vi "Do snap rpc cmd.vi"(8 "error in (no error)":errorcluster, 9 "Custom Command":string, 10 "Radio Address":string) -> (0 "error out":errorcluster, 1 "Cmd":string, 2 "standard error":string, 3 "trimmed string":string, 4 "return code":i32, 5 "standard output":string, 6 "Data item 1":string, 7 "Real volts":dbl, 11 "State":bool)   [LabVIEW 2013]
uses:
  1000336 func types.ctl
panel:
  in  "Function":T1
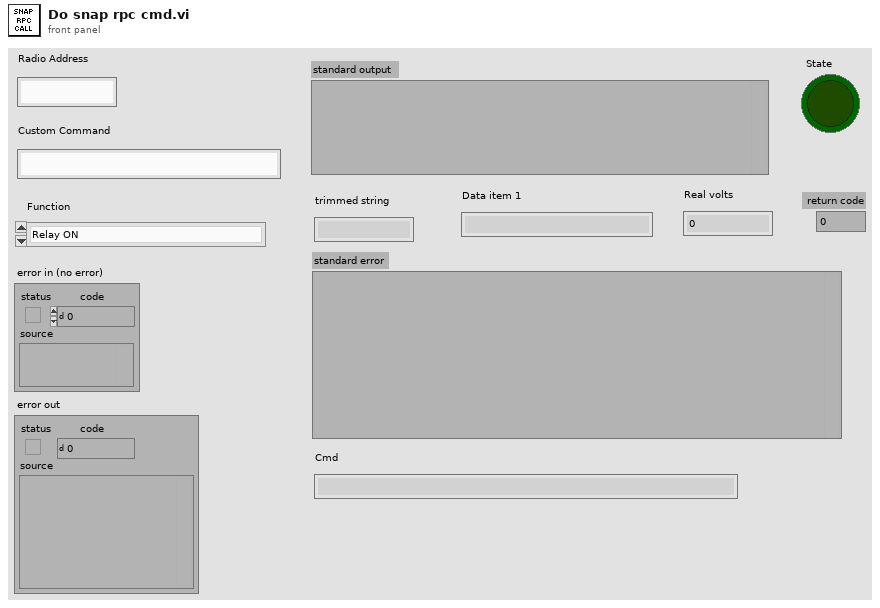
[diagram p1: front panel]
types:
  T1 = typedef "1000336 func types.ctl" = enum16{"Relay ON", "Relay OFF", "Override switch ON?", "Override switch OFF?", "Meas_vdc", "Meas_24v", "Meas_3.3v", "Blue led ON", "Blue led OFF", "Red led ON", "Red led OFF", "Green led ON", "Green led OFF", "Auto led ON", "Auto led OFF", "Custom cmd", "Get relay state", "Get major software version", "Get minor software version", "Get build version"}
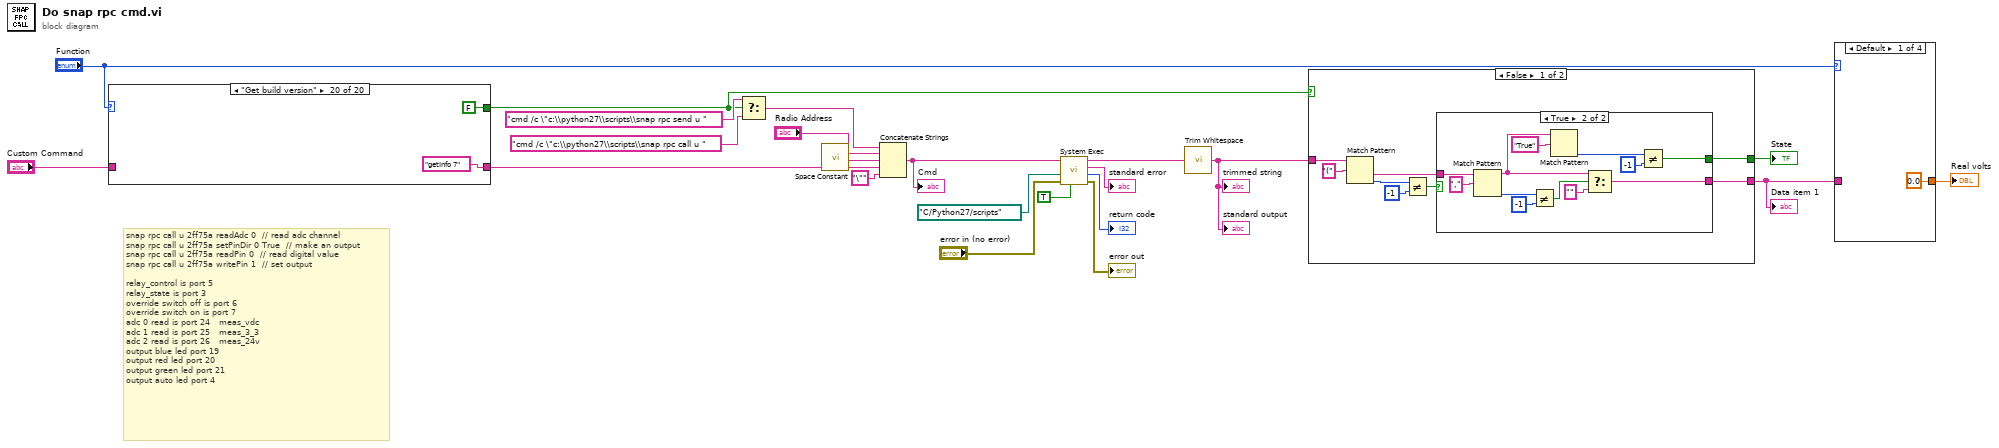
[diagram p0: block diagram]
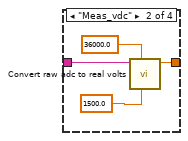
[diagram p2: hidden frame]
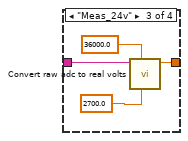
[diagram p3: hidden frame]
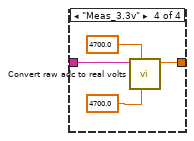
[diagram p4: hidden frame]
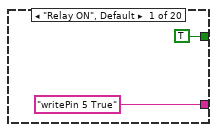
[diagram p5: hidden frame]
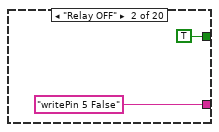
[diagram p6: hidden frame]
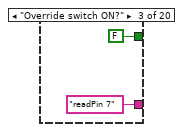
[diagram p7: hidden frame]
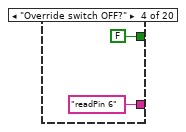
[diagram p8: hidden frame]
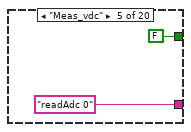
[diagram p9: hidden frame]
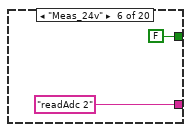
[diagram p10: hidden frame]
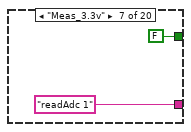
[diagram p11: hidden frame]
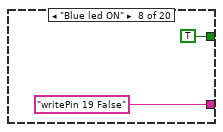
[diagram p12: hidden frame]
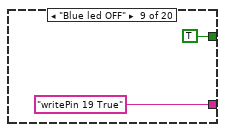
[diagram p13: hidden frame]
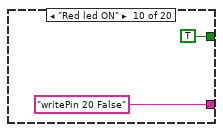
[diagram p14: hidden frame]
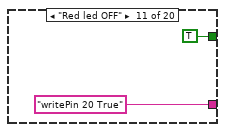
[diagram p15: hidden frame]
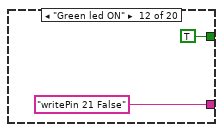
[diagram p16: hidden frame]
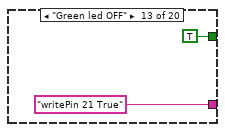
[diagram p17: hidden frame]
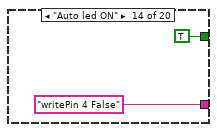
[diagram p18: hidden frame]
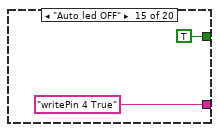
[diagram p19: hidden frame]
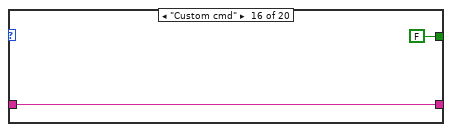
[diagram p20: hidden frame]
diagram:
  # "snap rpc call u 2ff75a readAdc 0\t\t// read adc channel\nsnap rpc call u 2ff75a setPinDir 0 True\t\t// make an output\nsnap rpc call u 2ff75a readPin 0\t\t// read digital value\nsnap rpc call u 2ff75a writePin 1\t\t// set output\n\nrelay_control is port 5\nrelay_state is port 3\noverride switch off is port 6\noverride switch on is port 7\nadc 0 read is port 24   meas_vdc\nadc 1 read is port 25   meas_3_3\nadc 2 read is port 26   meas_24v\noutput blue led port 19\noutput red led port 20\noutput green led port 21\noutput auto led port 4"
  n1 = case shown="\"Get build version\"" "Function" {
    tunnel: ["writePin 5 True" "writePin 5 False" "readPin 7" "readPin 6" "readAdc 0" "readAdc 2" "readAdc 1" "writePin 19 False" "writePin 19 True" "writePin 20 False" "writePin 20 True" "writePin 21 False" "writePin 21 True" "writePin 4 False" "writePin 4 True" w54 "readPin 3" ("Custom Command") "getInfo 5" ("Custom Command") "getInfo 6" ("Custom Command") "getInfo 7" ("Custom Command")] -> w7
    tunnel: "Custom Command" -> [_ _ _ _ _ _ _ _ _ _ _ _ _ _ _ w54 _ _ _ _]
    tunnel: [TRUE TRUE FALSE FALSE FALSE FALSE FALSE TRUE TRUE TRUE TRUE TRUE TRUE TRUE TRUE FALSE FALSE FALSE FALSE FALSE] -> w3
    frame "Relay ON", Default {
    }
    frame "Relay OFF" {
    }
    frame "Override switch ON?" {
    }
    frame "Override switch OFF?" {
    }
    frame "Meas_vdc" {
    }
    frame "Meas_24v" {
    }
    frame "Meas_3.3v" {
    }
    frame "Blue led ON" {
    }
    frame "Blue led OFF" {
    }
    frame "Red led ON" {
    }
    frame "Red led OFF" {
    }
    frame "Green led ON" {
    }
    frame "Green led OFF" {
    }
    frame "Auto led ON" {
    }
    frame "Auto led OFF" {
    }
    frame "Custom cmd" {
    }
    frame "Get relay state" {
    }
    frame "Get major software version" {
    }
    frame "Get minor software version" {
    }
    frame "Get build version" {
    }
  }
  n2 = Select(t="cmd /c \"c:\\python27\\scripts\\snap rpc send u " ("command line"), s=w3, f="cmd /c \"c:\\python27\\scripts\\snap rpc call u " ("command line")) -> (s? t:f=w18:string)
  n3 = call <vilib>:"Space Constant.vi"() -> ("String"=w20:string)
  n4 = Concatenate Strings(w18, "Radio Address", w20, w7, "\"" ("string")) -> (w22:string)
  "Cmd" <- w22
  n5 = call <vilib>:"System Exec.vi"("run minimized? (F)"=TRUE, "error in (no error)"="error in (no error)", "working directory"=path "C:/Python27/scripts", "command line"=w22) -> ("error out"=→"error out":errorcluster, "return code"=→"return code":i32, "standard error"=→"standard error":string, "standard output"=w15:string)  [unwired: 4 in]
  n6 = call <vilib>:"Trim Whitespace.vi"("string"=w15) -> ("trimmed string"=w8:string)  [unwired: 1 in]
  "standard output" <- w8
  "trimmed string" <- w8
  n7 = case shown="False" w3 {
    tunnel: w8 -> [w70 w92]
    tunnel: [w64 w86] -> w2
    tunnel: [w63 w85] -> w5
    frame False {
      n8 = Match Pattern(string=w70, regular expression="(") -> (after substring=w65:string, offset past match=w68:i32)  [unwired: 1 in, 2 out]
      n9 = Not Equal?(x=w68, y=-1) -> (x != y?=w66:bool)
      n10 = case shown="True" w66 {
        tunnel: w65 -> [_ w84]
        tunnel: ["" ("f") w78] -> w64
        tunnel: [FALSE w73] -> w63
        frame False {
        }
        frame True {
          n11 = Match Pattern(string=w84, regular expression=",") -> (before substring=w74:string, offset past match=w81:i32)  [unwired: 1 in, 2 out]
          n12 = Not Equal?(x=w81, y=-1) -> (x != y?=w80:bool)
          n13 = Match Pattern(string=w74, regular expression="True") -> (offset past match=w76:i32)  [unwired: 1 in, 3 out]
          n14 = Select(t=w74, s=w80, f="") -> (s? t:f=w78:string)
          n15 = Not Equal?(x=w76, y=-1) -> (x != y?=w73:bool)
        }
      }
    }
    frame True {
      n16 = Match Pattern(string=w92, regular expression="True") -> (offset past match=w90:i32)  [unwired: 1 in, 3 out]
      n17 = Not Equal?(x=w90, y=-1) -> (x != y?=w85:bool)
      n18 = Select(t="True", s=w85, f="False") -> (s? t:f=w86:string)
    }
  }
  "Data item 1" <- w2
  "State" <- w5
  n19 = case shown="Default" "Function" {
    tunnel: w2 -> [_ w97 w99 w103]
    tunnel: [0.0 ("Real volts") w94 w98 w102] -> w1
    frame Default {
    }
    frame "Meas_vdc" {
      n20 = call "Convert raw adc to real volts.vi"("Lower resistor (none)"=1500.0, "Upper resistor (none)"=36000.0, "Raw ADC value"=w97) -> ("Real volts"=w94:dbl)  [unwired: 7 in, 1 out]
    }
    frame "Meas_24v" {
      n21 = call "Convert raw adc to real volts.vi"("Lower resistor (none)"=2700.0, "Upper resistor (none)"=36000.0, "Raw ADC value"=w99) -> ("Real volts"=w98:dbl)  [unwired: 7 in, 1 out]
    }
    frame "Meas_3.3v" {
      n22 = call "Convert raw adc to real volts.vi"("Lower resistor (none)"=4700.0, "Upper resistor (none)"=4700.0, "Raw ADC value"=w103) -> ("Real volts"=w102:dbl)  [unwired: 7 in, 1 out]
    }
  }
  "Real volts" <- w1
